vi "Autonomous.vi"   [LabVIEW 2017]
doc: "This VI starts when autonomous period begins, and will automatically be terminated when it ends. You can carry out timed or sensor driven operations directly to I/O or to subsystems without needing to return to the caller."
uses:
  <vilib>/Rock Robotics/Network Tables/NT Read String.vi
  <vilib>/Rock Robotics/WPI/Utilities/WPI_GetSetVariantRefNum.vi
  <vilib>/Rock Robotics/Network Tables/NT Read Number.vi
  <vilib>/Rock Robotics/Network Tables/NT Read Raw.vi
types:
  T1 = cluster{"Enable":bool, "Switch Left":bool, "Scale Left":bool}
  T2 = typedef "WPI_JoystickDevRef.ctl" = cluster{"Device":T3}
  T3 = typedef "WPI_JoystickDeviceEnum.ctl" = enum16{"USB 0", "USB 1", "USB 2", "USB 3", "USB 4", "USB 5"}
  T4 = typedef "Command Status Info.ctl" = cluster{"Name":string, "Status":T5, "notifier out":T6}
  T5 = typedef "Completion Status.ctl" = enum16{"Successful", "Aborted", "Incomplete"}
  T6 = typedef "Completion Notifier.ctl" = refnum<notifier>
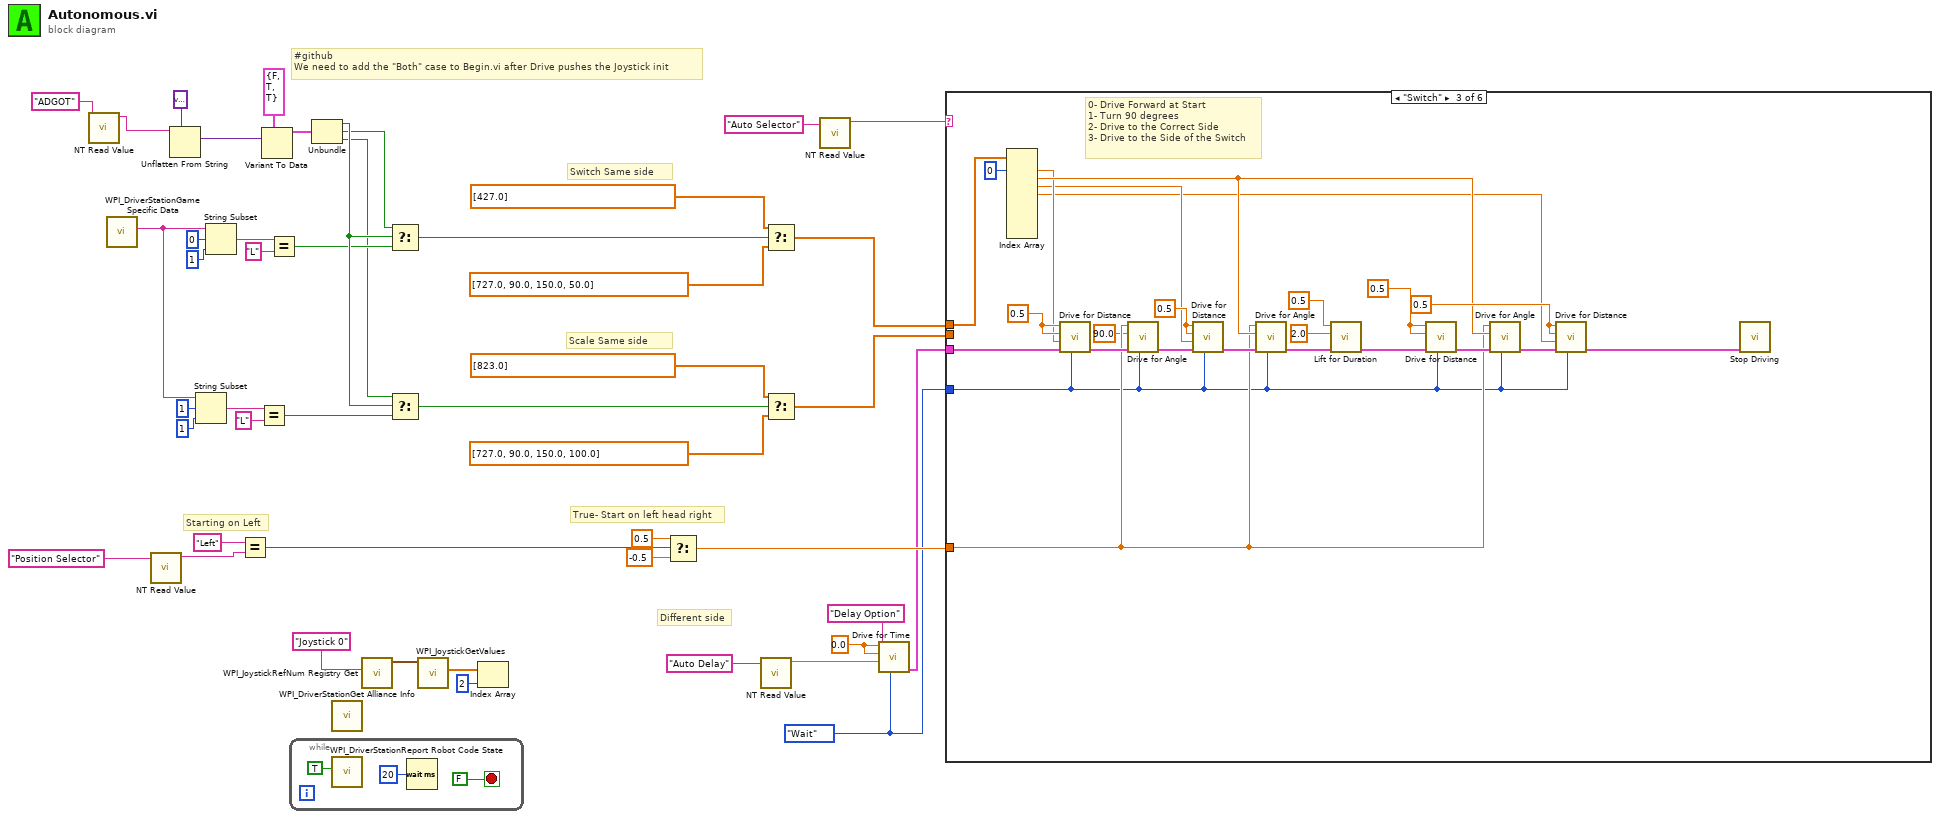
[diagram p0: block diagram]
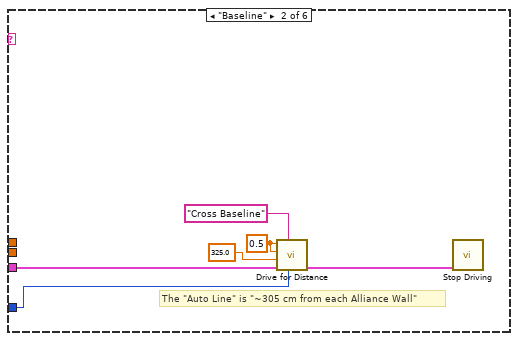
[diagram p3: hidden frame]
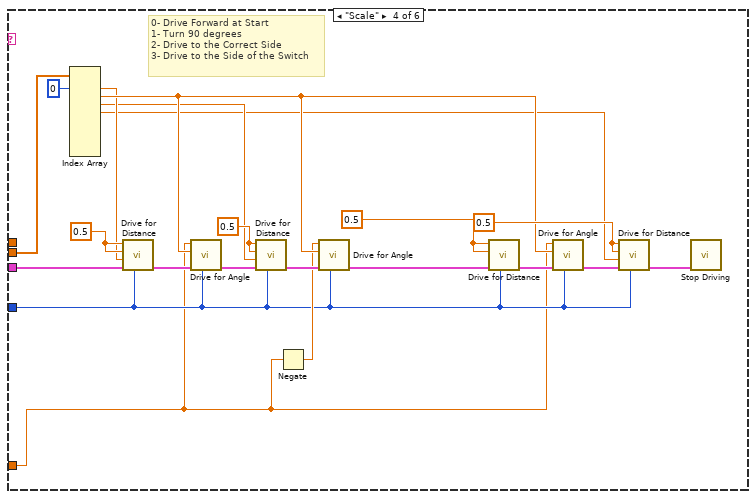
[diagram p4: hidden frame]
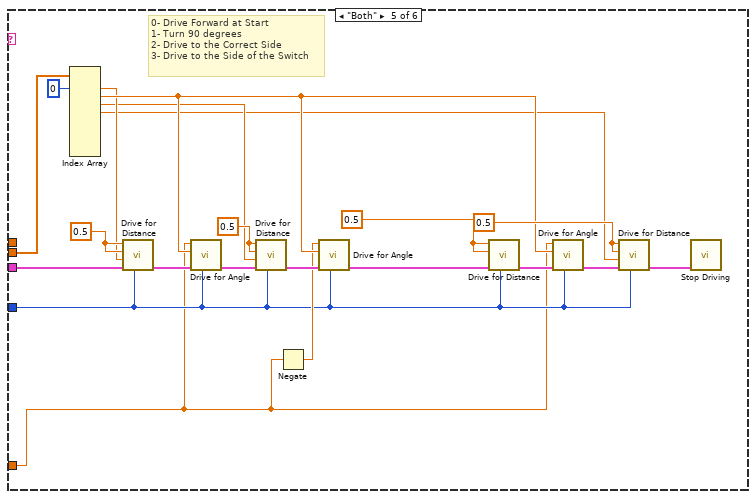
[diagram p5: hidden frame]
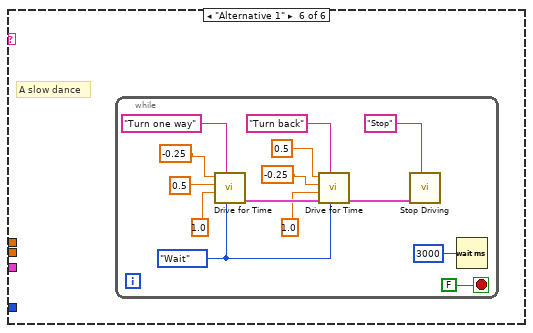
[diagram p6: hidden frame]
diagram:
  w18 = enum16{"Start", "Wait"}."Wait" ("Synchronication")
  w17 = 0.0 ("Left Speed")
  # "#github \nWe need to add the \"Both\" case to Begin.vi after Drive pushes the Joystick init"
  # "Different side"
  # "Scale Same side"
  # "Starting on Left"
  # "True- Start on left head right"
  # "Switch Same side"
  n1 = call-poly <vilib>:"NT Read Value.vi"("Name"="ADGOT") -> ("Raw"=w12:string)  [unwired: 9 in, 1 out]
  n2 = call <vilib>:"WPI_DriverStationGame Specific Data.vi"() -> ("Game Specific Data"=w28:string)  [unwired: 11 in]
  n3 = call-poly <vilib>:"NT Read Value.vi"("Name"="Position Selector") -> ("String"=w22:string)  [unwired: 9 in, 1 out]
  n4 = Unflatten From String(type=variant, binary string=w12) -> (value=w10:variant)  [unwired: 3 in, 2 out]
  n5 = String Subset(string=w28, offset (0)=1, length (rest)=1 ("length (rest)")) -> (substring=w29:string)
  n6 = String Subset(string=w28, offset (0)=0, length (rest)=1 ("length (rest)")) -> (substring=w39:string)
  n7 = Equal?(x="Left", y=w22) -> (x = y?=w14:bool)
  n8 = Equal?(x=w29, y="L") -> (x = y?=w6:bool)
  n9 = Variant To Data(type=T1 {"Enable"=FALSE, "Switch Left"=TRUE, "Scale Left"=TRUE} ("Auton Game Data Override for Testing"), Variant=w10) -> (data=w8:T1)  [unwired: 1 in, 1 out]
  n10 = Equal?(x=w39, y="L") -> (x = y?=w5:bool)
  n11 = while {
    stop <- FALSE stop-if-true
    n12 = call <vilib>:"WPI_DriverStationReport Robot Code State.vi"("Autonomous"=TRUE) -> ()  [unwired: 10 in, 1 out]
    n13 = Wait (ms)(milliseconds to wait=u32 20) -> ()  [unwired: 1 out]
  }
  n14 = Unbundle(w8) -> ("Enable"=w7:bool, "Switch Left"=w4:bool, "Scale Left"=w3:bool)
  n15 = call <vilib>:"WPI_DriverStationGet Alliance Info.vi"() -> ()  [unwired: 12 out]
  n16 = call <vilib>:"WPI_JoystickRefNum Registry Get.vi"("refnum name"="Joystick 0") -> ("JoystickDevRef"=w43:T2)  [unwired: 1 in, 9 out]
  n17 = Select(t=w4, s=w7, f=w5) -> (s? t:f=w2:bool)
  n18 = Select(t=w3, s=w7, f=w6) -> (s? t:f=w1:bool)
  n19 = call <vilib>:"WPI_JoystickGetValues.vi"("JoystickDevRef"=w43) -> ("Axes"=w42:dbl[])  [unwired: 6 in, 4 out]
  n20 = Index Array(array=w42, index=2) -> ()  [unwired: 1 out]
  n21 = Select(t=0.5, s=w14, f=-0.5) -> (s? t:f=w33:dbl)
  n22 = call-poly <vilib>:"NT Read Value.vi"("Name"="Auto Delay") -> ("Numeric"=w15:dbl)  [unwired: 9 in, 1 out]
  n23 = Select(t=dbl[] [427.0], s=w2, f=dbl[] [727.0, 90.0, 150.0, 50.0]) -> (s? t:f=w36:dbl[])
  n24 = Select(t=dbl[] [823.0], s=w1, f=dbl[] [727.0, 90.0, 150.0, 100.0]) -> (s? t:f=w25:dbl[])
  n25 = call-poly <vilib>:"NT Read Value.vi"("Name"="Auto Selector") -> ("String"=w16:string)  [unwired: 9 in, 1 out]
  n26 = call "Drive for Time.vi"("Synchronization"=w18, "Description"="Delay Option", "Seconds"=w15, "Right Speed"=w17, "Left Speed"=w17) -> ("Command Info Out"=w19:T4)  [unwired: 5 in, 1 out]
  n27 = case shown="\"Switch\"" w16 {
    tunnel: w36 -> [_ _ w71 _ _ _]
    tunnel: w33 -> [_ _ w68 w81 w102 _]
    tunnel: w25 -> [_ _ _ w85 w106 _]
    tunnel: w19 -> [_ w55 w62 w83 w104 _]
    tunnel: w18 -> [_ w52 w61 w82 w103 _]
    frame "Nothing", Default {
    }
    frame "Baseline" {
      w54 = 0.5 ("Left Setpoint")
      # "The \"Auto Line\" is \"~305 cm from each Alliance Wall\""
      n28 = call "Drive for Distance.vi"("Synchronication"=w52, "Description"="Cross Baseline", "Command Info In"=w55, "Distance"=325.0, "Right Setpoint"=w54, "Left Setpoint"=w54) -> ("Command Info Out"=w56:T4)  [unwired: 5 in]
      n29 = call "Stop Driving.vi"("Command Info In"=w56) -> ()  [unwired: 10 in, 1 out]
    }
    frame "Switch" {
      w72 = 0.5 ("Left Setpoint")
      w73 = 0.5 ("Left Setpoint")
      w74 = 0.5 ("Left Setpoint")
      w75 = 0.5 ("Left Setpoint")
      # "0- Drive Forward at Start\n1- Turn 90 degrees\n2- Drive to the Correct Side\n3- Drive to the Side of the Switch"
      n30 = Index Array(array=w71, index #1=0) -> (element #1=w67:dbl, element #2=w69:dbl, element #3=w66:dbl, element #4=w65:dbl)  [unwired: 8 in, 5 out]
      n31 = call "Drive for Distance.vi"("Synchronication"=w61, "Command Info In"=w62, "Distance"=w67, "Right Setpoint"=w75, "Left Setpoint"=w75) -> ("Command Info Out"=w80:T4)  [unwired: 6 in]
      n32 = call "Drive for Angle.vi"("Synchronication"=w61, "Command Info In"=w80, "Angle"=90.0, "Setpoint"=w68) -> ("Command Info Out"=w79:T4)  [unwired: 7 in]
      n33 = call "Drive for Distance.vi"("Synchronication"=w61, "Command Info In"=w79, "Distance"=w66, "Right Setpoint"=w74, "Left Setpoint"=w74) -> ("Command Info Out"=w78:T4)  [unwired: 6 in]
      n34 = call "Drive for Angle.vi"("Synchronication"=w61, "Command Info In"=w78, "Angle"=w69, "Setpoint"=w68) -> ("Command Info Out"=w58:T4)  [unwired: 7 in]
      n35 = call "Lift for Duration.vi"("Command Info In"=w58, "Duration (s)"=2.0, "Setpoint"=0.5) -> ("Command Info Out"=w59:T4)  [unwired: 8 in]
      n36 = call "Drive for Distance.vi"("Synchronication"=w61, "Command Info In"=w59, "Right Setpoint"=w73, "Left Setpoint"=w73) -> ("Command Info Out"=w77:T4)  [unwired: 7 in]
      n37 = call "Drive for Angle.vi"("Synchronication"=w61, "Command Info In"=w77, "Angle"=w69, "Setpoint"=w68) -> ("Command Info Out"=w76:T4)  [unwired: 7 in]
      n38 = call "Drive for Distance.vi"("Synchronication"=w61, "Command Info In"=w76, "Distance"=w65, "Right Setpoint"=w72, "Left Setpoint"=w72) -> ("Command Info Out"=w64:T4)  [unwired: 6 in]
      n39 = call "Stop Driving.vi"("Command Info In"=w64) -> ()  [unwired: 10 in, 1 out]
    }
    frame "Scale" {
      w92 = 0.5 ("Left Setpoint")
      w93 = 0.5 ("Left Setpoint")
      w94 = 0.5 ("Left Setpoint")
      w95 = 0.5 ("Left Setpoint")
      # "0- Drive Forward at Start\n1- Turn 90 degrees\n2- Drive to the Correct Side\n3- Drive to the Side of the Switch"
      n40 = Index Array(array=w85, index #1=0) -> (element #1=w89:dbl, element #2=w90:dbl, element #3=w88:dbl, element #4=w87:dbl)  [unwired: 8 in, 5 out]
      n41 = call "Drive for Distance.vi"("Synchronication"=w82, "Command Info In"=w83, "Distance"=w89, "Right Setpoint"=w95, "Left Setpoint"=w95) -> ("Command Info Out"=w101:T4)  [unwired: 6 in]
      n42 = call "Drive for Angle.vi"("Synchronication"=w82, "Command Info In"=w101, "Angle"=w90, "Setpoint"=w81) -> ("Command Info Out"=w100:T4)  [unwired: 7 in]
      n43 = call "Drive for Distance.vi"("Synchronication"=w82, "Command Info In"=w100, "Distance"=w88, "Right Setpoint"=w94, "Left Setpoint"=w94) -> ("Command Info Out"=w99:T4)  [unwired: 6 in]
      n44 = Negate(x=w81) -> (-x=w84:dbl)
      n45 = call "Drive for Angle.vi"("Synchronication"=w82, "Command Info In"=w99, "Angle"=w90, "Setpoint"=w84) -> ("Command Info Out"=w98:T4)  [unwired: 7 in]
      n46 = call "Drive for Distance.vi"("Synchronication"=w82, "Command Info In"=w98, "Right Setpoint"=w93, "Left Setpoint"=w93) -> ("Command Info Out"=w97:T4)  [unwired: 7 in]
      n47 = call "Drive for Angle.vi"("Synchronication"=w82, "Command Info In"=w97, "Angle"=w90, "Setpoint"=w81) -> ("Command Info Out"=w96:T4)  [unwired: 7 in]
      n48 = call "Drive for Distance.vi"("Synchronication"=w82, "Command Info In"=w96, "Distance"=w87, "Right Setpoint"=w92, "Left Setpoint"=w92) -> ("Command Info Out"=w86:T4)  [unwired: 6 in]
      n49 = call "Stop Driving.vi"("Command Info In"=w86) -> ()  [unwired: 10 in, 1 out]
    }
    frame "Both" {
      w113 = 0.5 ("Left Setpoint")
      w114 = 0.5 ("Left Setpoint")
      w115 = 0.5 ("Left Setpoint")
      w116 = 0.5 ("Left Setpoint")
      # "0- Drive Forward at Start\n1- Turn 90 degrees\n2- Drive to the Correct Side\n3- Drive to the Side of the Switch"
      n50 = Index Array(array=w106, index #1=0) -> (element #1=w110:dbl, element #2=w111:dbl, element #3=w109:dbl, element #4=w108:dbl)  [unwired: 8 in, 5 out]
      n51 = call "Drive for Distance.vi"("Synchronication"=w103, "Command Info In"=w104, "Distance"=w110, "Right Setpoint"=w116, "Left Setpoint"=w116) -> ("Command Info Out"=w122:T4)  [unwired: 6 in]
      n52 = call "Drive for Angle.vi"("Synchronication"=w103, "Command Info In"=w122, "Angle"=w111, "Setpoint"=w102) -> ("Command Info Out"=w121:T4)  [unwired: 7 in]
      n53 = call "Drive for Distance.vi"("Synchronication"=w103, "Command Info In"=w121, "Distance"=w109, "Right Setpoint"=w115, "Left Setpoint"=w115) -> ("Command Info Out"=w120:T4)  [unwired: 6 in]
      n54 = Negate(x=w102) -> (-x=w105:dbl)
      n55 = call "Drive for Angle.vi"("Synchronication"=w103, "Command Info In"=w120, "Angle"=w111, "Setpoint"=w105) -> ("Command Info Out"=w119:T4)  [unwired: 7 in]
      n56 = call "Drive for Distance.vi"("Synchronication"=w103, "Command Info In"=w119, "Right Setpoint"=w114, "Left Setpoint"=w114) -> ("Command Info Out"=w118:T4)  [unwired: 7 in]
      n57 = call "Drive for Angle.vi"("Synchronication"=w103, "Command Info In"=w118, "Angle"=w111, "Setpoint"=w102) -> ("Command Info Out"=w117:T4)  [unwired: 7 in]
      n58 = call "Drive for Distance.vi"("Synchronication"=w103, "Command Info In"=w117, "Distance"=w108, "Right Setpoint"=w113, "Left Setpoint"=w113) -> ("Command Info Out"=w107:T4)  [unwired: 6 in]
      n59 = call "Stop Driving.vi"("Command Info In"=w107) -> ()  [unwired: 10 in, 1 out]
    }
    frame "Alternative 1" {
      # "A slow dance"
      n60 = while {
        stop <- FALSE stop-if-true
        w127 = enum16{"Start", "Wait"}."Wait" ("Synchronication")
        n61 = call "Drive for Time.vi"("Synchronization"=w127, "Description"="Turn one way", "Seconds"=1.0 ("Delay (s)"), "Right Speed"=0.5 ("X axis value"), "Left Speed"=-0.25 ("X axis value")) -> ("Command Info Out"=w136:T4)  [unwired: 5 in, 1 out]
        n62 = call "Drive for Time.vi"("Synchronization"=w127, "Description"="Turn back", "Command Info In"=w136, "Seconds"=1.0 ("Delay (s)"), "Right Speed"=-0.25 ("X axis value"), "Left Speed"=0.5 ("X axis value")) -> ("Command Info Out"=w126:T4)  [unwired: 4 in, 1 out]
        n63 = call "Stop Driving.vi"("Description"="Stop", "Command Info In"=w126) -> ()  [unwired: 9 in, 1 out]
        n64 = Wait (ms)(milliseconds to wait=u32 3000 ("millisecond timer value")) -> ()  [unwired: 1 out]
      }
    }
  }
